vi "rqcBob Key Distribution (Low Level Example).vi"() -> ()   [LabVIEW 2018]
uses:
  Custom Controls/rqcBob States.ctl
  FPGA/rqcBob/Custom Controls/rqcBob Trigger Type.ctl
  Shared/Shared FPGA Lib/Shared Logic/Custom Controls/rqc Random Generator.parameters.ctl
  Shared/Shared FPGA Lib/Shared Logic/Custom Controls/rqc Random Generator.value type.ctl
  FPGA/rqcBob/Custom Controls/rqcBob Window Config.ctl
  FPGA/rqcBob/Custom Controls/rqcBob Modulator Config.ctl
  FPGA/rqcBob/Custom Controls/Pulse Train/rqcBob Pulse Train Config.ctl
  FPGA/rqcBob/Custom Controls/Pulse Train/rqcBob Pulse Train.Generation Mode.ctl
  FPGA/rqcBob/Custom Controls/Pulse Train/rqcBob Pulse Train.First Pulse Delay Mode.ctl
  Shared/Shared Host Lib/rqc ServiceNET/Custom Controls/rqc ServiceNET command.ctl
  Shared/Shared Host Lib/rqc ServiceNET/Bob/Custom Controls/rqcBob ServiceNET control.ctl
  <vilib>/FPGAPlugInAG/PCI-7811R/niLvFpga_Open_PCI-7811R.vi
  <vilib>/rvi/interface/common/dynamic/niFpgaDynamicAddResources.vi
  Low Level API/Configuration/Photon Detector/Set PD window/rqcBob Configure SPD Detection Window (2PD).vi
  Shared/Shared Host Lib/rqc ServiceNET/Bob/rqcBob Send Data/rqcBob ServiceNET Send Data U32.vi
  Shared/Shared Host Lib/rqc ServiceNET/Bob/rqcBob Send Data/rqcBob ServiceNET Send Data U8.vi
  <vilib>/FPGAPlugInAG/Dynamic/niLvFpga_Close_Dynamic.vi
  <vilib>/rvi/interface/nirviOpenFPGA/nirviOpenFPGA.xnode
  FPGA Bitfiles/rqcBob (FPGA) 7811 v 4.0.0.lvbitx
  <vilib>/rvi/interface/nirviCloseFPGA/nirviCloseFPGA.xnode
panel:
  in  "Activate advanced parameters":bool
  in  "Autoscale X":bool=TRUE caption="Show all mesurements"
  out "current States":T1=enum."App.Stop" caption="App current state"
  in  "Number of States":enum32{"2 Random States", "4 Random States"}(radio)=enum."4 Random States"
  out "Key length graph":i32(graph)
  in  "Modulator shift":fxp<+,4,4>=3.0
  in  "Check D2":u8 caption="D2 window"
  in  "Random\nOn/Off":bool=TRUE caption="Bob's states\nrandomisation"
  in  "Pi Voltage":u16
  in  "Number of trains":u16
  in  "Number of pulses in train":u16
  in  "Train Period":u16
  in  "Open window":u16 caption="Detection starts at\n(in units of 200 ns)"
  out "Key length (s)":i32 caption="Bob key length, bits"
  out "Bob's Key:":string
  out "Incorrect Alice's data":bool
  out "Total pulses expected:":u32
  in  "Data shift":u8=3 max=7 step=1
  out "error out":errorcluster
  out "Connected to Alice":bool caption="Connection status"
  in  "Stop":bool
  in  "Check D1":u8 caption="D1 window"
  in  "Port:":u16=5020
  in  "Alice's IP address":string="10.32.64.203"
  # "FPGA settings:"
  # "BOB"
  # "LAN settings:"
  # "Advanced Parameters"
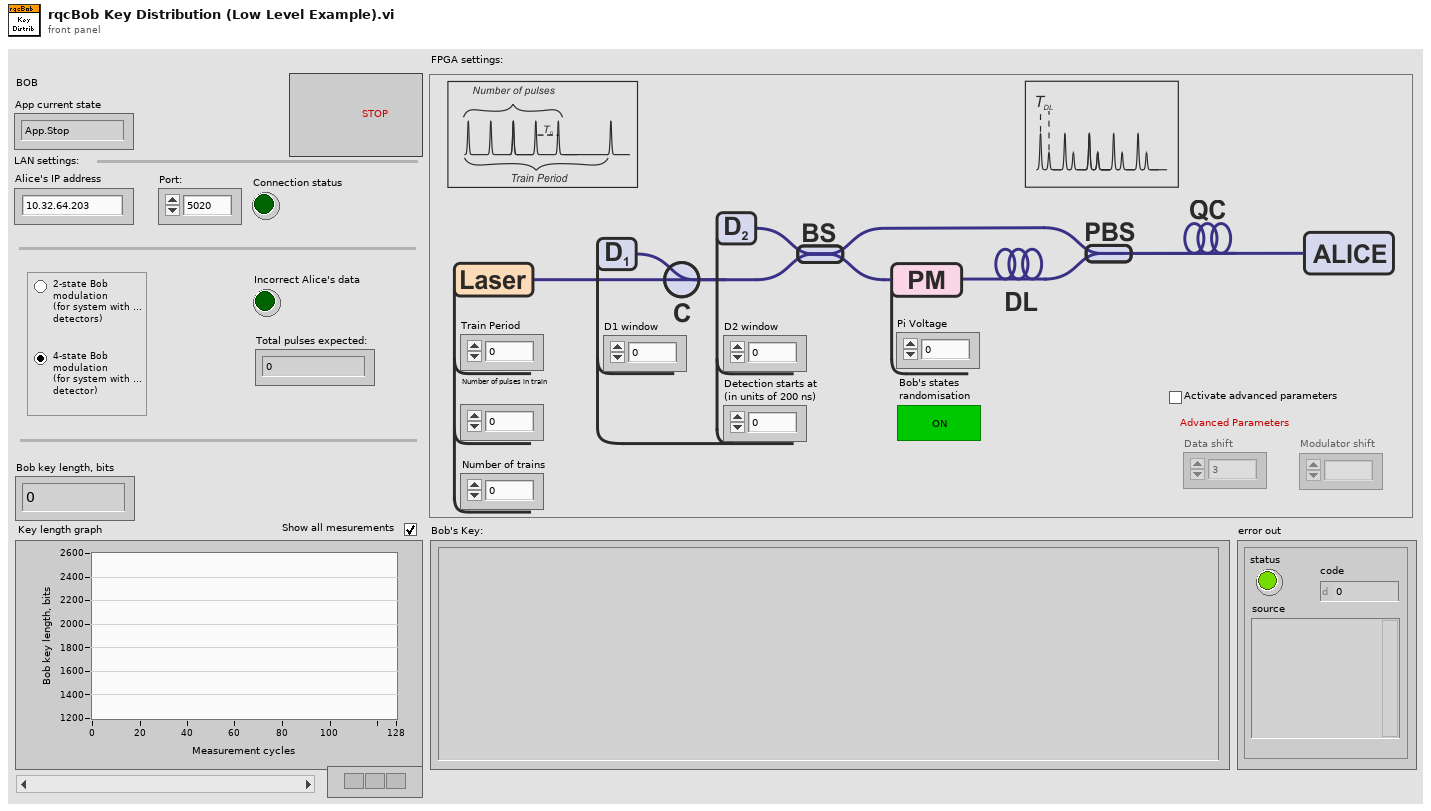
[diagram p1: front panel]
types:
  T1 = typedef "rqcBob States.ctl" = enum16{"HW.configure", "HW.sendTrigger", "HW.initiate", "HW.measure", "HW.stop", "NET.create", "NET.connect", "NET.sendCommand", "NET.readCommand", "NET.readData", "NET.close", "App.HandleEvent", "App.HandleError", "App.Stop"}
  T2 = typedef "rqcBob Trigger Type.ctl" = enum16{"software", "immediate", "DIO"}
  T3 = typedef "rqcBob Pulse Train Config.ctl" = cluster{"period":u16, "num of pulses":u16, "mode":T4, "num of trains":u16, "first pulse delay mode":T5, "first pulse delay":u16}
  T4 = typedef "rqcBob Pulse Train.Generation Mode.ctl" = enum32{"single train", "train sequence.single", "train sequence.wait for trigger", "continuous"}
  T5 = typedef "rqcBob Pulse Train.First Pulse Delay Mode.ctl" = enum8{"none", "every train", "first train"}
  T6 = typedef "rqcBob Modulator Config.ctl" = cluster{"modulator.start":u16, "modulator.stop":u16}
  T7 = typedef "rqcBob Window Config.ctl" = cluster{"window.open":u16, "window.close":u16}
  T8 = typedef "rqc Random Generator.parameters.ctl" = cluster{"value type":T9, "constant":u16, "num of levels":u16, "levels values":u16[]}
  T9 = typedef "rqc Random Generator.value type.ctl" = enum32{"random value", "constant"}
  T10 = typedef "rqc ServiceNET command.ctl" = enum8{"NONE", "READY", "START", "PING"}
  T11 = typedef "rqcBob ServiceNET control.ctl" = cluster{"connection ID":refnum<k5>, "connected?":bool, "Alice's IP address":string, "port":u16}
  T12 = enum8{"Enabled", "Disabled", "Disabled and Grayed Out"}
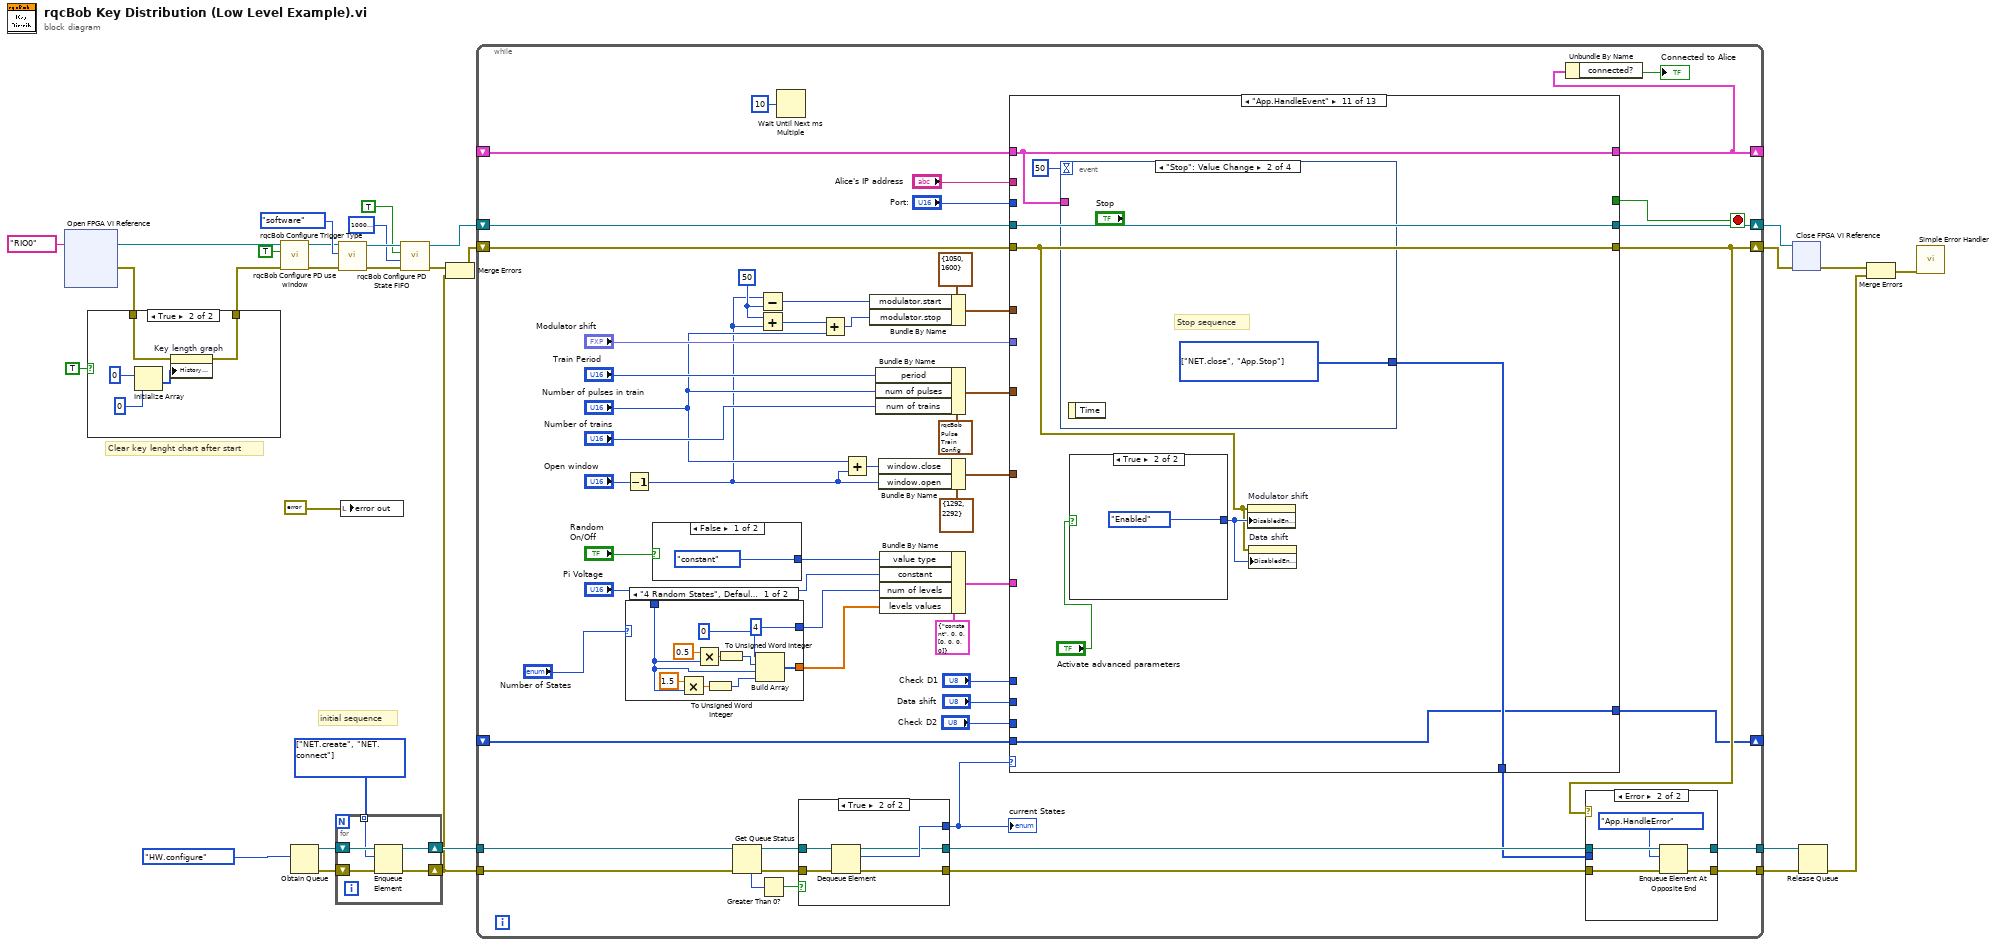
[diagram p0: block diagram]
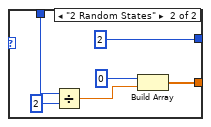
[diagram p3: hidden frame]
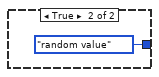
[diagram p4: hidden frame]
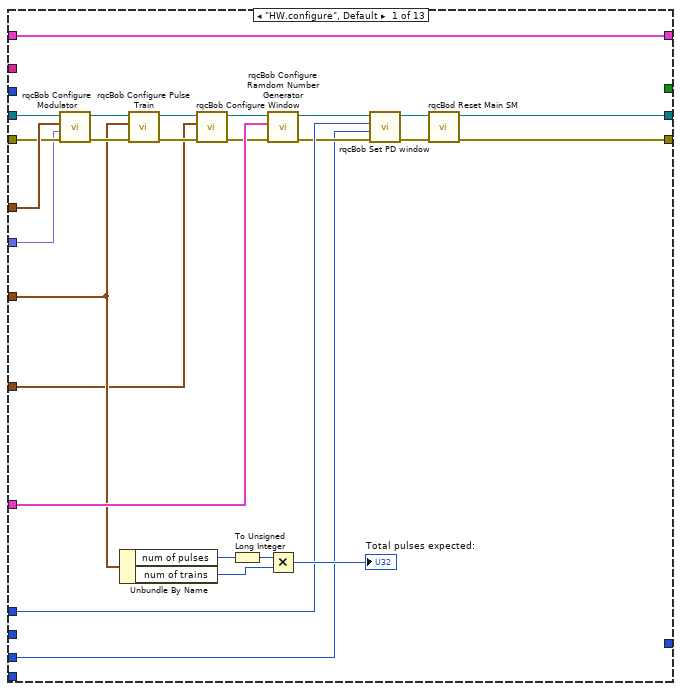
[diagram p5: hidden frame]
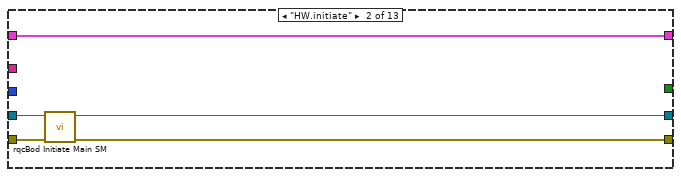
[diagram p6: hidden frame]
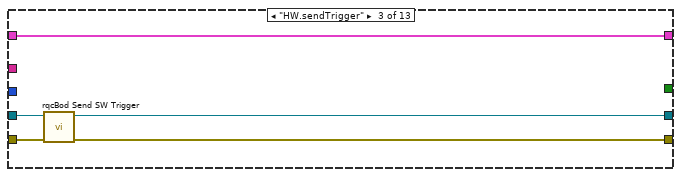
[diagram p7: hidden frame]
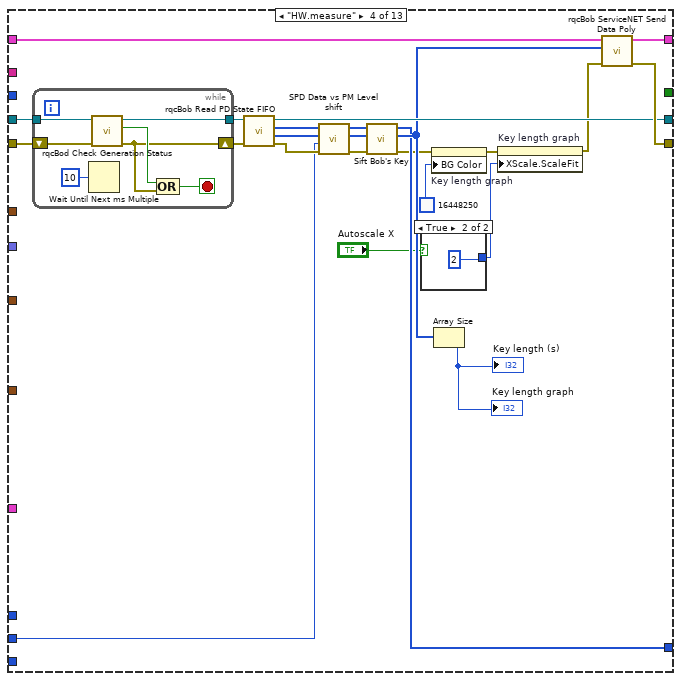
[diagram p8: hidden frame]
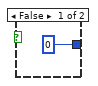
[diagram p9: hidden frame]
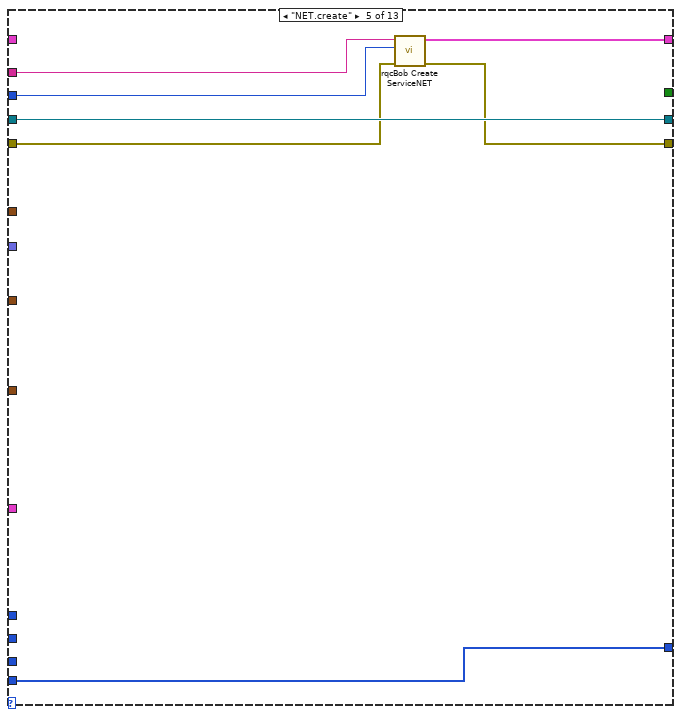
[diagram p10: hidden frame]
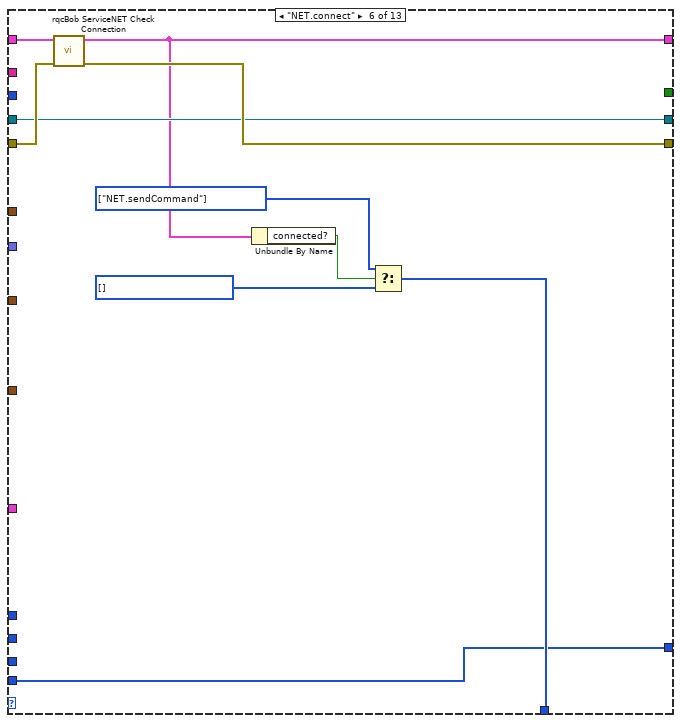
[diagram p11: hidden frame]
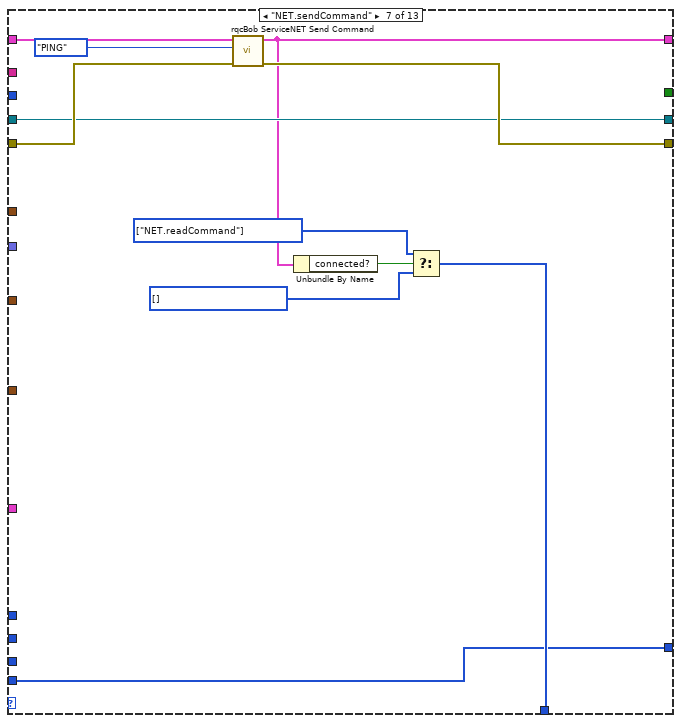
[diagram p12: hidden frame]
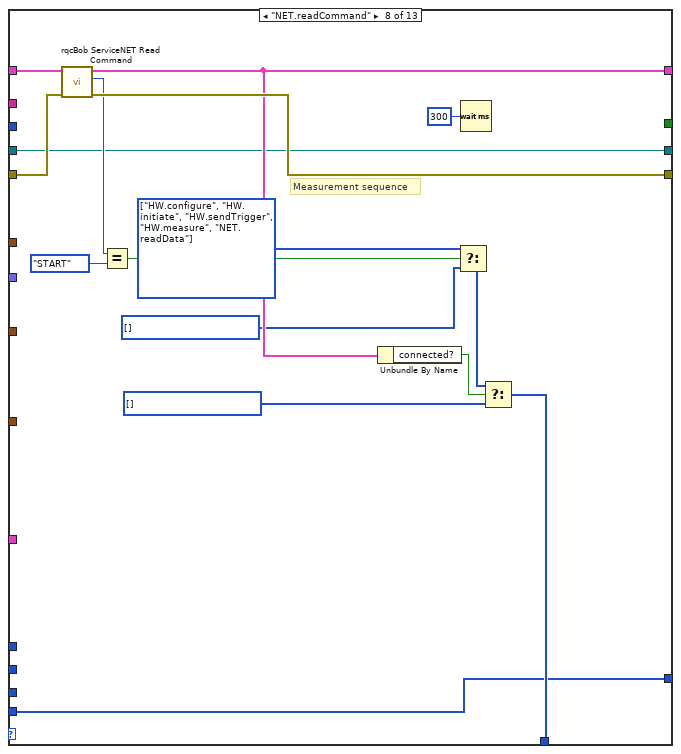
[diagram p13: hidden frame]
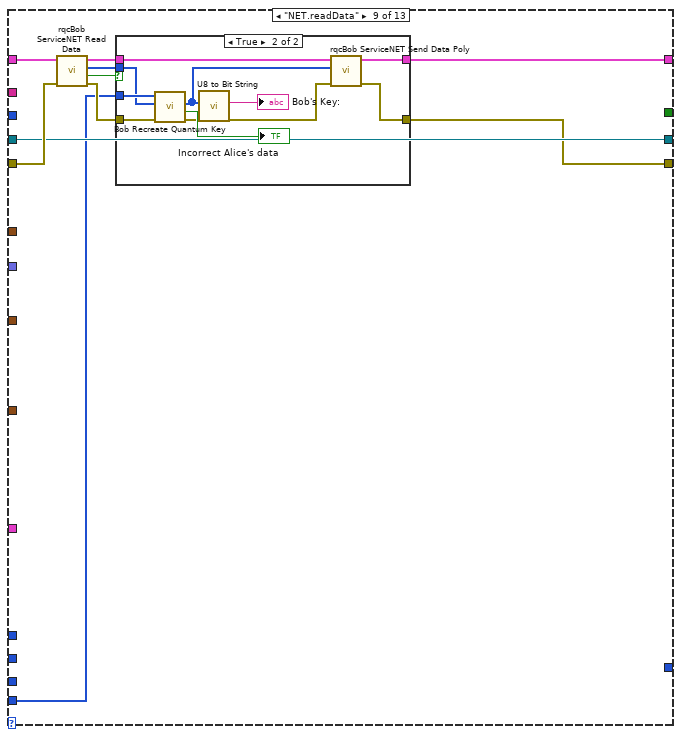
[diagram p14: hidden frame]
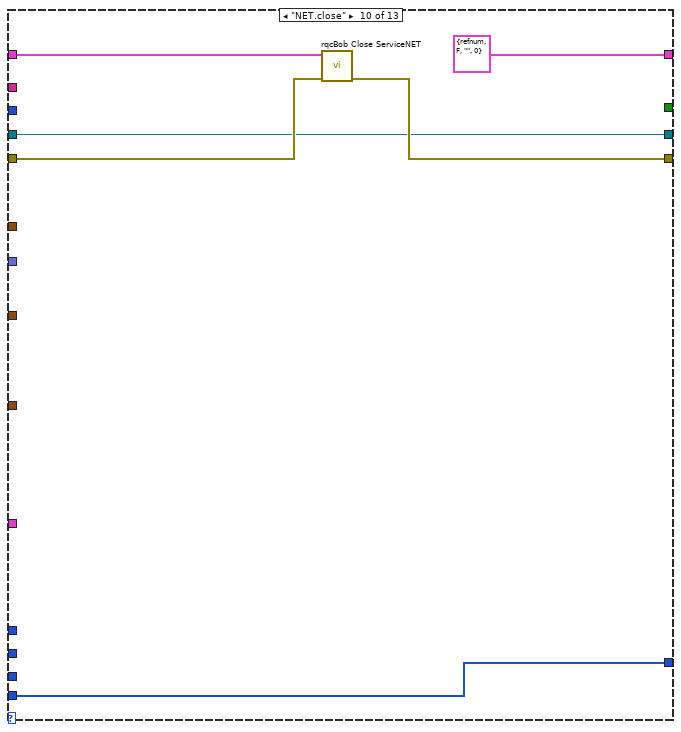
[diagram p16: hidden frame]
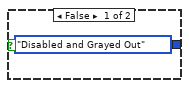
[diagram p17: hidden frame]
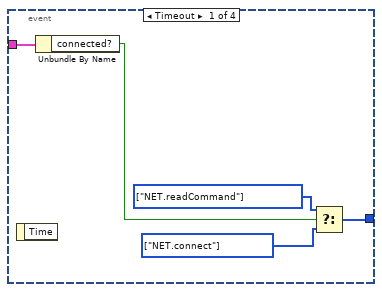
[diagram p18: hidden frame]
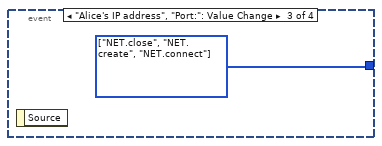
[diagram p19: hidden frame]
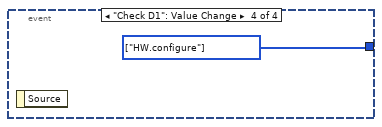
[diagram p20: hidden frame]
diagram:
  w24 = T1[] [enum."NET.create", enum."NET.connect"] items=["HW.configure", "HW.sendTrigger", "HW.initiate", "HW.measure", "HW.stop", "NET.create", "NET.connect", "NET.sendCommand", "NET.readCommand", "NET.readData", "NET.close", "App.HandleEvent", "App.HandleError", "App.Stop"]
  # "Clear key lenght chart after start"
  # "initial sequence"
  n1 = xnode "Open FPGA VI Reference"("resource name"=tag "RIO0") -> ("FPGA VI Reference Out"=w8:refnum<k20>, "error out"=w3:errorcluster)  [unwired: 1 in]
  n2 = case shown="True" TRUE {
    tunnel: w3 -> [w31 w36]
    tunnel: [w31 w35] -> w2
    frame False {
    }
    frame True {
      n3 = Initialize Array(0 ("element"), 0 ("dimension size")) -> (w34:i32[])
      n4 = property on="Key length graph" class="WFChart (strict)"(error in=w36, "History Data"=w34) -> (error out=w35:errorcluster)  [unwired: 1 in, 1 out]
    }
  }
  n5 = call "rqcBob Configure PD use window.vi"("error in"=w2, "PD.use window"=TRUE, "FPGA reference in"=w8) -> ("error out"=w6:errorcluster, "FPGA reference out"=w7:refnum<k20>)  [unwired: 7 in]
  n6 = Obtain Queue(element data type=rqcBob_States."HW.configure" ("rqcBob States")) -> (queue out=w29:refnum<queue>, error out=w28:errorcluster)  [unwired: 4 in, 1 out]
  n7 = for {
    tunnel: w24 -> [w37] mode=indexing
    shift-right: [w38] -> w26
    shift-left: w29 -> [w41]
    shift-right: [w39] -> w23
    shift-left: w28 -> [w40]
    n8 = Enqueue Element(queue=w41, element=w37, error in (no error)=w40) -> (queue out=w38:refnum<queue>, error out=w39:errorcluster)  [unwired: 1 in, 1 out]
  }
  n9 = call "rqcBob Configure Trigger Type.vi"("error in"=w6, "rqcBob Trigger Type"=rqcBob_Trigger_Type."software", "FPGA reference in"=w7) -> ("error out"=w11:errorcluster, "FPGA reference out"=w14:refnum<k20>)  [unwired: 7 in]
  n10 = local write "error out"(errorcluster {"status"=FALSE, "code"=0, "source"=""} ("error constant")) -> ()
  n11 = call "rqcBob Configure PD State FIFO.vi"("error in"=w11, "PD.state fifo depth"=u32 10000000 ("SPD.detect fifo depth"), "PD.state fifo write enable"=TRUE ("SPD.detect fifo write enable"), "FPGA reference in"=w14) -> ("error out"=w12:errorcluster, "FPGA reference out"=w13:refnum<k20>)  [unwired: 6 in]
  n12 = Merge Errors(w12, w23) -> (w27:errorcluster)
  n13 = while {
    shift-right: [w78] -> w22
    shift-left: w27 -> [w89]
    shift-right: [w79] -> w21
    shift-left: w13 -> [w76]
    tunnel: w26 -> [w87]
    tunnel: w23 -> [w86]
    tunnel: [w81] -> w20
    tunnel: [w80] -> w19
    shift-right: [w72] -> _
    shift-left: _ -> [w73]
    shift-right: [w68] -> _
    shift-left: _ -> [w67]
    stop <- w77 stop-if-true
    w60 = 50
    n14 = Decrement(x="Open window") -> (x-1=w44:u16)
    n15 = case shown="\"4 Random States\", Default" "Number of States" {
      tunnel: [w95 w110] -> w52
      tunnel: [u16 4 ("pm.DAC num of levels") u16 2 ("pm.DAC num of levels")] -> w51
      tunnel: "Pi Voltage" -> [w96 w107]
      frame "4 Random States", Default {
        n16 = Multiply(x=1.5, y=w96) -> (x*y=w101:dbl)
        n17 = Multiply(x=0.5, y=w96) -> (x*y=w103:dbl)
        n18 = To Unsigned Word Integer(number=w101) -> (unsigned 16bit integer=w98:u16)
        n19 = To Unsigned Word Integer(number=w103) -> (unsigned 16bit integer=w99:u16)
        n20 = Build Array(u16 0, w99, w96, w98) -> (w95:u16[])
      }
      frame "2 Random States" {
        n21 = Divide(x=w107, y=u16 2) -> (x/y=w106:dbl)
        n22 = Build Array(u16 0, w106) -> (w110:dbl[])
      }
    }
    n23 = case shown="False" "Random\nOn/Off" {
      tunnel: [rqc_Random_Generator.value_type."constant" ("value type") rqc_Random_Generator.value_type."random value" ("value type")] -> w53
      frame False {
      }
      frame True {
      }
    }
    n24 = Get Queue Status(queue=w87, error in (no error)=w86) -> (queue out=w83:refnum<queue>, error out=w82:errorcluster, # elements in queue=w85:i32)  [unwired: 1 in, 5 out]
    n25 = Subtract(x=w44, y=w60) -> (x-y=w57:i32)
    n26 = Add(x=w60, y=w44) -> (x+y=w56:i32)
    n27 = Greater Than 0?(x=w85) -> (x > 0?=w84:bool)
    n28 = Wait Until Next ms Multiple(millisecond multiple=u32 10) -> ()  [unwired: 1 out]
    n29 = case shown="True" w84 {
      tunnel: w83 -> [w283 w290]
      tunnel: w82 -> [w284 w289]
      tunnel: [rqcBob_States."App.HandleEvent" ("rqcBob States") w288] -> w42
      tunnel: [w283 w287] -> w91
      tunnel: [w284 w286] -> w88
      frame False {
      }
      frame True {
        n30 = Dequeue Element(queue=w290, error in (no error)=w289) -> (queue out=w287:refnum<queue>, element=w288:T1, error out=w286:errorcluster)  [unwired: 1 in, 1 out]
      }
    }
    "current States" <- w42
    n31 = Add(x=w56, y="Number of pulses in train") -> (x+y=w55:i32)
    n32 = Add(x="Number of pulses in train", y=w44) -> (x+y=w48:u16)
    n33 = Bundle By Name(cluster=T6 {"modulator.start"=1050, "modulator.stop"=1600} ("modulator.config"), "modulator.start"=w57, "modulator.stop"=w55) -> (w58:T6)
    n34 = Bundle By Name(cluster=T3 {"period"=4000, "num of pulses"=1000, "mode"=enum."train sequence.single", "num of trains"=1000, "first pulse delay mode"=enum."every train", "first pulse delay"=55} ("train.configuration"), "period"="Train Period", "num of pulses"="Number of pulses in train", "num of trains"="Number of trains") -> (w65:T3)
    n35 = Bundle By Name(cluster=T7 {"window.open"=1292, "window.close"=2292} ("window.config"), "window.close"=w48, "window.open"=w44) -> (w66:T7)
    n36 = Bundle By Name(cluster=T8 {"value type"=enum."constant", "constant"=0, "num of levels"=0, "levels values"=[0, 0, 0, 0]} ("rqcBob rndGen.parameters"), "value type"=w53, "constant"="Pi Voltage", "num of levels"=w51, "levels values"=w52) -> (w63:T8)
    n37 = case shown="\"App.HandleEvent\"" w42 {
      tunnel: w58 -> [w138 _ _ _ _ _ _ _ _ _ _ _ _]
      tunnel: w65 -> [w121 _ _ _ _ _ _ _ _ _ _ _ _]
      tunnel: w66 -> [w114 _ _ _ _ _ _ _ _ _ _ _ _]
      tunnel: w63 -> [w125 _ _ _ _ _ _ _ _ _ _ _ _]
      tunnel: "Check D1" -> [w128 _ _ _ _ _ _ _ _ _ _ _ _]
      tunnel: [w134 w140 w145 w169 w183 w196 w207 w223 w229 w250 w254 errorcluster {"status"=FALSE, "code"=0, "source"=""} ("error constant") w280] -> w78
      tunnel: w89 -> [w137 w142 w147 w149 w184 w197 w208 w224 w234 w251 w254 w275 w280]
      tunnel: [_ _ _ _ _ w190 w200 w219 _ _ w259 w274 _] -> w90
      tunnel: [w135 w141 w146 w166 w188 w195 w206 w212 w233 w249 w260 w277 w281] -> w79
      tunnel: [_ _ _ _ _ _ _ _ _ _ _ FALSE TRUE] -> w77
      tunnel: w76 -> [w136 w143 w148 w172 w188 w195 w206 w212 w233 w249 w260 w277 w281]
      tunnel: "Alice's IP address" -> [_ _ _ _ w187 _ _ _ _ _ _ _ _]
      tunnel: "Port:" -> [_ _ _ _ w186 _ _ _ _ _ _ _ _]
      tunnel: [w133 w139 w144 w171 w185 w194 w204 w220 w227 T11 {"connection ID"=refnum, "connected?"=FALSE, "Alice's IP address"="", "port"=0} ("rqcBob ServiceNET control") w258 w276 w279] -> w72
      tunnel: w73 -> [w133 w139 w144 w170 _ w198 w209 w225 w235 w253 w258 w276 w279]
      tunnel: "Data shift" -> [_ _ _ w161 _ _ _ _ _ _ _ _ _]
      tunnel: [_ _ _ w157 w182 w189 w199 w211 _ w248 w257 _ _] -> w68
      tunnel: w67 -> [_ _ _ _ w182 w189 w199 w211 w226 w248 w257 _ _]
      tunnel: "Modulator shift" -> [w124 _ _ _ _ _ _ _ _ _ _ _ _]
      tunnel: "Check D2" -> [w113 _ _ _ _ _ _ _ _ _ _ _ _]
      frame "HW.configure", Default {
        n38 = call "rqcBob Configure Modulator.vi"("error in"=w137, "modulator.clock delay"=w124, "modulator.config"=w138, "FPGA reference in"=w136) -> ("error out"=w122:errorcluster, "FPGA reference out"=w123:refnum<k20>)  [unwired: 6 in]
        n39 = Unbundle By Name(w121) -> ("num of pulses"=w131:u16, "num of trains"=w130:u16)
        n40 = call "rqcBob Configure Pulse Train.vi"("error in"=w122, "train.configuration"=w121, "FPGA reference in"=w123) -> ("error out"=w118:errorcluster, "FPGA reference out"=w119:refnum<k20>)  [unwired: 6 in, 1 out]
        n41 = call "rqcBob Configure Window.vi"("error in"=w118, "window.config"=w114, "FPGA reference in"=w119) -> ("error out"=w117:errorcluster, "FPGA reference out"=w120:refnum<k20>)  [unwired: 7 in]
        n42 = To Unsigned Long Integer(number=w131) -> (unsigned 32bit integer=w129:u32)
        n43 = call "rqcBob Configure Ramdom Number Generator.vi"("error in"=w117, "rqcBob rndGen.parameters"=w125, "FPGA reference in"=w120) -> ("error out"=w126:errorcluster, "FPGA reference out"=w127:refnum<k20>)  [unwired: 7 in]
        n44 = Multiply(x=w129, y=w130) -> (x*y=→"Total pulses expected:":u32)
        n45 = call-poly "rqcBob Set PD window.vi"("error in"=w126, "PD2.detection window"=w113, "PD1.detection window"=w128, "FPGA reference in"=w127) -> ("error out"=w116:errorcluster, "FPGA reference out"=w115:refnum<k20>)  [unwired: 6 in]
        n46 = call "rqcBod Reset Main SM.vi"("error in"=w116, "FPGA reference in"=w115) -> ("error out"=w134:errorcluster, "FPGA reference out"=w135:refnum<k20>)  [unwired: 8 in]
      }
      frame "HW.initiate" {
        n47 = call "rqcBod Initiate Main SM.vi"("error in"=w142, "FPGA reference in"=w143) -> ("error out"=w140:errorcluster, "FPGA reference out"=w141:refnum<k20>)  [unwired: 8 in]
      }
      frame "HW.sendTrigger" {
        n48 = call "rqcBod Send SW Trigger.vi"("error in"=w147, "FPGA reference in"=w148) -> ("error out"=w145:errorcluster, "FPGA reference out"=w146:refnum<k20>)  [unwired: 8 in]
      }
      frame "HW.measure" {
        n49 = while {
          tunnel: w172 -> [w181]
          shift-right: [w175] -> w167
          shift-left: w149 -> [w180]
          tunnel: [w177] -> w168
          stop <- w176 stop-if-true
          n50 = Wait Until Next ms Multiple(millisecond multiple=u32 10) -> ()  [unwired: 1 out]
          n51 = call "rqcBod Check Generation Status.vi"("error in"=w180, "FPGA reference in"=w181) -> ("error out"=w175:errorcluster, "generation.done"=w178:bool, "FPGA reference out"=w177:refnum<k20>)  [unwired: 7 in]
          n52 = Compound Arithmetic op=OR(w178, w175) -> (w176:bool)
        }
        n53 = call "rqcBob Read PD State FIFO.vi"("error in"=w167, "FPGA reference in"=w168) -> ("error out"=w162:errorcluster, "PM Level"=w159:u8[], "SPD Number"=w160:u8[], "FPGA reference out"=w166:refnum<k20>)  [unwired: 6 in]
        n54 = call "SPD Data vs PM Level shift.vi"("error in"=w162, "Data shift"=w161, "PM Level in"=w159, "SPD Number in"=w160) -> ("error out"=w165:errorcluster, "PM Level out"=w163:u8[], "SPD Number out"=w164:u8[])  [unwired: 5 in]
        n55 = call "Sift Bob's Key.vi"("error in"=w165, "PM Level in"=w163, "SPD Number in"=w164) -> ("error out"=w155:errorcluster, "Sifted Bob's data"=w158:u32[], "Raw Bob's data"=w157:u8[])  [unwired: 6 in]
        n56 = case shown="True" "Autoscale X" {
          tunnel: [u8 0 u8 2] -> w151
          frame False {
          }
          frame True {
          }
        }
        n57 = property on="Key length graph" class="WFChart (strict)"(error in=w155, "BG Color"=u32 16448250) -> (error out=w154:errorcluster)  [unwired: 1 in, 1 out]
        n58 = Array Size(array=w158) -> (size(s)=→"Key length (s)" →"Key length graph":i32)
        n59 = property on="Key length graph" class="WFChart (strict)"(error in=w154, "XScale.ScaleFit"=w151) -> (error out=w153:errorcluster)  [unwired: 1 in, 1 out]
        n60 = call-poly "rqcBob ServiceNET Send Data Poly.vi"("error in"=w153, "Data"=w158, "rqcBob ServiceNET in"=w170) -> ("error out"=w169:errorcluster, "rqcBob ServiceNET out"=w171:T11)  [unwired: 7 in]
      }
      frame "NET.create" {
        n61 = call "rqcBob Create ServiceNET.vi"("error in"=w184, "port"=w186, "Alice's IP address"=w187) -> ("error out"=w183:errorcluster, "rqcBob ServiceNET control"=w185:T11)  [unwired: 7 in]
      }
      frame "NET.connect" {
        w191 = T1[] [] items=["HW.configure", "HW.sendTrigger", "HW.initiate", "HW.measure", "HW.stop", "NET.create", "NET.connect", "NET.sendCommand", "NET.readCommand", "NET.readData", "NET.close", "App.HandleEvent", "App.HandleError", "App.Stop"] ("f")
        w193 = T1[] [enum."NET.sendCommand"] items=["HW.configure", "HW.sendTrigger", "HW.initiate", "HW.measure", "HW.stop", "NET.create", "NET.connect", "NET.sendCommand", "NET.readCommand", "NET.readData", "NET.close", "App.HandleEvent", "App.HandleError", "App.Stop"]
        n62 = call "rqcBob ServiceNET Check Connection.vi"("error in"=w197, "rqcBob ServiceNET in"=w198) -> ("error out"=w196:errorcluster, "rqcBob ServiceNET out"=w194:T11)  [unwired: 8 in]
        n63 = Unbundle By Name(w194) -> ("connected?"=w192:bool)
        n64 = Select(t=w193, s=w192, f=w191) -> (s? t:f=w190:T1[])
      }
      frame "NET.sendCommand" {
        w201 = T1[] [] items=["HW.configure", "HW.sendTrigger", "HW.initiate", "HW.measure", "HW.stop", "NET.create", "NET.connect", "NET.sendCommand", "NET.readCommand", "NET.readData", "NET.close", "App.HandleEvent", "App.HandleError", "App.Stop"] ("f")
        w202 = T1[] [enum."NET.readCommand"] items=["HW.configure", "HW.sendTrigger", "HW.initiate", "HW.measure", "HW.stop", "NET.create", "NET.connect", "NET.sendCommand", "NET.readCommand", "NET.readData", "NET.close", "App.HandleEvent", "App.HandleError", "App.Stop"] ("f")
        n65 = call "rqcBob ServiceNET Send Command.vi"("error in"=w208, "command"=rqc_ServiceNET_command."PING", "rqcBob ServiceNET in"=w209) -> ("error out"=w207:errorcluster, "rqcBob ServiceNET out"=w204:T11)  [unwired: 7 in]
        n66 = Unbundle By Name(w204) -> ("connected?"=w203:bool)
        n67 = Select(t=w202, s=w203, f=w201) -> (s? t:f=w200:T1[])
      }
      frame "NET.readCommand" {
        w214 = T1[] [] items=["HW.configure", "HW.sendTrigger", "HW.initiate", "HW.measure", "HW.stop", "NET.create", "NET.connect", "NET.sendCommand", "NET.readCommand", "NET.readData", "NET.close", "App.HandleEvent", "App.HandleError", "App.Stop"] ("f")
        w221 = T1[] [] items=["HW.configure", "HW.sendTrigger", "HW.initiate", "HW.measure", "HW.stop", "NET.create", "NET.connect", "NET.sendCommand", "NET.readCommand", "NET.readData", "NET.close", "App.HandleEvent", "App.HandleError", "App.Stop"] ("f")
        w215 = T1[] [enum."HW.configure", enum."HW.initiate", enum."HW.sendTrigger", enum."HW.measure", enum."NET.readData"] items=["HW.configure", "HW.sendTrigger", "HW.initiate", "HW.measure", "HW.stop", "NET.create", "NET.connect", "NET.sendCommand", "NET.readCommand", "NET.readData", "NET.close", "App.HandleEvent", "App.HandleError", "App.Stop"] ("f")
        # "Measurement sequence"
        n68 = call "rqcBob ServiceNET Read Command.vi"("error in"=w224, "rqcBob ServiceNET in"=w225) -> ("error out"=w223:errorcluster, "command"=w218:T10, "rqcBob ServiceNET out"=w220:T11)  [unwired: 6 in, 1 out]
        n69 = Equal?(x=w218, y=rqc_ServiceNET_command."START") -> (x = y?=w216:bool)
        n70 = Unbundle By Name(w220) -> ("connected?"=w222:bool)
        n71 = Select(t=w215, s=w216, f=w214) -> (s? t:f=w213:T1[])
        n72 = Wait (ms)(milliseconds to wait=u32 300) -> ()  [unwired: 1 out]
        n73 = Select(t=w213, s=w222, f=w221) -> (s? t:f=w219:T1[])
      }
      frame "NET.readData" {
        n74 = call "rqcBob ServiceNET Read Data.vi"("error in"=w234, "rqcBob ServiceNET in"=w235) -> ("error out"=w231:errorcluster, "data valid"=w230:bool, "Data"=w232:u32[], "rqcBob ServiceNET out"=w228:T11)  [unwired: 6 in]
        n75 = case shown="True" w230 {
          tunnel: w226 -> [_ w247]
          tunnel: w232 -> [_ w246]
          tunnel: w231 -> [w237 w245]
          tunnel: [w237 w241] -> w229
          tunnel: w228 -> [w236 w243]
          tunnel: [w236 w242] -> w227
          frame False {
          }
          frame True {
            n76 = call "Bob Recreate Quantum Key.vi"("error in"=w245, "Correct Measurements Indexes in"=w246, "Raw Data in"=w247) -> ("error out"=w238:errorcluster, "Incorrect Alice's data"=→"Incorrect Alice's data":bool, "Sifted Key out"=w240:u8[])  [unwired: 6 in]
            n77 = call "U8 to Bit String.vi"("U8 in"=w240) -> ("String out"=→"Bob's Key:":string)  [unwired: 10 in]
            n78 = call-poly "rqcBob ServiceNET Send Data Poly.vi"("error in"=w238, "Data"=w240, "rqcBob ServiceNET in"=w243) -> ("error out"=w241:errorcluster, "rqcBob ServiceNET out"=w242:T11)  [unwired: 7 in]
          }
        }
      }
      frame "NET.close" {
        n79 = call "rqcBob Close ServiceNET.vi"("error in"=w251, "rqcBob ServiceNET control"=w253) -> ("error out"=w250:errorcluster)  [unwired: 9 in]
      }
      frame "App.HandleEvent" {
        n80 = event shown="[1] \"Stop\": Value Change" {
          selector: _ -> [_ _ _ _]
          dyn-events: _ -> [_ _ _ _]
          timeout: 50 -> [_ _ _ _]
          tunnel: [w267 w269 w270 w271] -> w259
          tunnel: w258 -> [w268 _ _ _]
          event Timeout {
            w264 = T1[] [enum."NET.connect"] items=["HW.configure", "HW.sendTrigger", "HW.initiate", "HW.measure", "HW.stop", "NET.create", "NET.connect", "NET.sendCommand", "NET.readCommand", "NET.readData", "NET.close", "App.HandleEvent", "App.HandleError", "App.Stop"]
            w265 = T1[] [enum."NET.readCommand"] items=["HW.configure", "HW.sendTrigger", "HW.initiate", "HW.measure", "HW.stop", "NET.create", "NET.connect", "NET.sendCommand", "NET.readCommand", "NET.readData", "NET.close", "App.HandleEvent", "App.HandleError", "App.Stop"]
            n81 = event-data() -> ()  [unwired: 1 in, 1 out]
            n82 = Unbundle By Name(w268) -> ("connected?"=w266:bool)
            n83 = Select(t=w265, s=w266, f=w264) -> (s? t:f=w267:T1[])
          }
          event "Stop": Value Change {
            w269 = T1[] [enum."NET.close", enum."App.Stop"] items=["HW.configure", "HW.sendTrigger", "HW.initiate", "HW.measure", "HW.stop", "NET.create", "NET.connect", "NET.sendCommand", "NET.readCommand", "NET.readData", "NET.close", "App.HandleEvent", "App.HandleError", "App.Stop"]
            # "Stop sequence"
            n84 = event-data() -> ()  [unwired: 1 in, 1 out]
          }
          event "Alice's IP address", "Port:": Value Change {
            w270 = T1[] [enum."NET.close", enum."NET.create", enum."NET.connect"] items=["HW.configure", "HW.sendTrigger", "HW.initiate", "HW.measure", "HW.stop", "NET.create", "NET.connect", "NET.sendCommand", "NET.readCommand", "NET.readData", "NET.close", "App.HandleEvent", "App.HandleError", "App.Stop"]
            n85 = event-data() -> ()  [unwired: 1 in, 1 out]
          }
          event "Check D1": Value Change {
            w271 = T1[] [enum."HW.configure"] items=["HW.configure", "HW.sendTrigger", "HW.initiate", "HW.measure", "HW.stop", "NET.create", "NET.connect", "NET.sendCommand", "NET.readCommand", "NET.readData", "NET.close", "App.HandleEvent", "App.HandleError", "App.Stop"]
            n86 = event-data() -> ()  [unwired: 1 in, 1 out]
          }
        }
        n87 = case shown="True" "Activate advanced parameters" {
          tunnel: [T12."Disabled and Grayed Out" ("Disabled") T12."Enabled" ("Disabled")] -> w256
          frame False {
          }
          frame True {
          }
        }
        n88 = property on="Modulator shift" class="DigNum (strict)"(error in=w254, "DisabledEnum"=w256) -> ()  [unwired: 1 in, 2 out]
        n89 = property on="Data shift" class="DigNum (strict)"(error in=w254, "DisabledEnum"=w256) -> ()  [unwired: 1 in, 2 out]
      }
      frame "App.HandleError" {
        # "Handle known ERRORS here"
        n90 = call "rqcBob Error Handler.vi"("error in (no error)"=w275, "rqcBob ServiceNET control"=w276) -> ("error out"=→"error out":errorcluster, "error sequence"=w274:T1[])  [unwired: 8 in]
      }
      frame "App.Stop" {
      }
    }
    n91 = Unbundle By Name(w72) -> ("connected?"=→"Connected to Alice":bool)
    n92 = case shown="Error" w78 {
      tunnel: w91 -> [w295 w305]
      tunnel: w90 -> [w292 _]
      tunnel: w88 -> [w291 w304]
      tunnel: [w294 w302] -> w81
      tunnel: [w293 w301] -> w80
      frame No Error {
        n93 = for {
          tunnel: w292 -> [w299] mode=indexing
          shift-right: [w297] -> w293
          shift-left: w291 -> [w298]
          shift-right: [w296] -> w294
          shift-left: w295 -> [w300]
          n94 = Enqueue Element(queue=w300, element=w299, error in (no error)=w298) -> (queue out=w296:refnum<queue>, error out=w297:errorcluster)  [unwired: 1 in, 1 out]
        }
      }
      frame Error {
        n95 = Enqueue Element At Opposite End(queue=w305, element=rqcBob_States."App.HandleError", error in (no error)=w304) -> (queue out=w302:refnum<queue>, error out=w301:errorcluster)  [unwired: 1 in, 1 out]
      }
    }
  }
  n96 = xnode "Close FPGA VI Reference"("FPGA VI Reference In"=w21, "error in"=w22) -> ("error out"=w18:errorcluster)
  n97 = Release Queue(queue=w20, error in (no error)=w19) -> (error out=w17:errorcluster)  [unwired: 1 in, 2 out]
  n98 = Merge Errors(w18, w17) -> (w16:errorcluster)
  n99 = call <vilib>:"Simple Error Handler.vi"("error in (no error)"=w16) -> ()  [unwired: 4 in, 5 out]
